vi "fun_Adjust waveform t0.vi"(8 "error in (no error)":errorcluster, 9 "delta Timestamp(ticks)":u64, 10 "waveform (Y)":waveform(dbl)[](array[waveform]), 11 "Handle In":T1 {"Handle" format="0x%08x"; "Conn" format="0x%08x"}) -> (0 "error out":errorcluster, 2 "Adjusted Waveform":waveform(dbl)[](array[waveform]), 3 "Handle Out":T1 {"Handle" format="0x%08x"; "Conn" format="0x%08x"})   [LabVIEW 2016]
uses:
  <instrlib>/Zurich Instruments LabOne/Public/ziTypeHandle.ctl
  <instrlib>/Zurich Instruments LabOne/Public/Utility/ziTicksToS_single.vi
  <instrlib>/Zurich Instruments LabOne/Zurich Instruments LabOne.lvlib
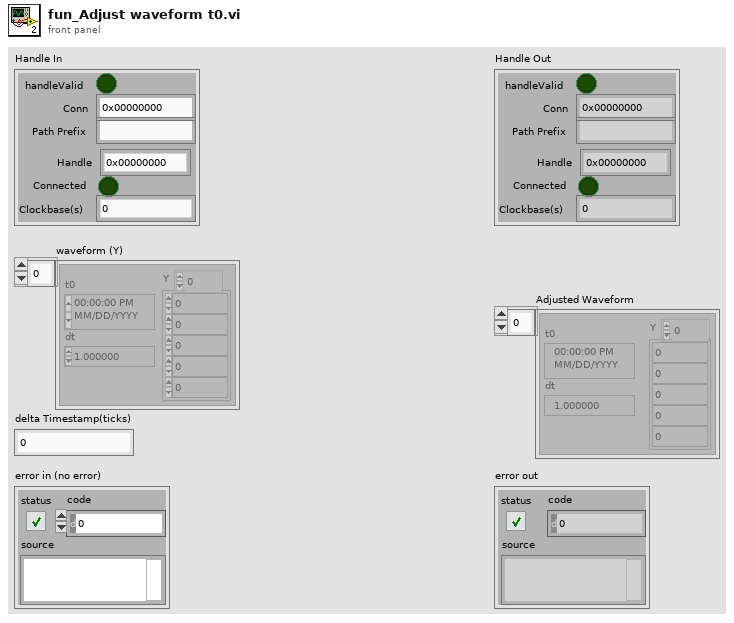
[diagram p1: front panel]
types:
  T1 = typedef "Zurich Instruments LabOne.lvlib/ziTypeHandle.ctl" = cluster{"handleValid":bool, "Conn":u64, "Path Prefix":string, "Handle":u64, "Connected":bool, "Clockbase(s)":dbl}
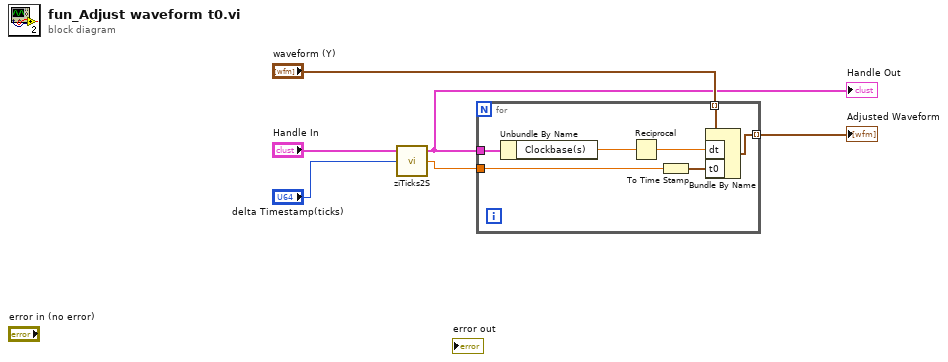
[diagram p0: block diagram]
diagram:
  n1 = call-poly <instrlib>:"ziTicks2S.vi"("Timestamp(ticks)"="delta Timestamp(ticks)", "Handle In"="Handle In") -> ("Timestamp(s)"=w1:dbl, "Handle Out"=w3:T1)  [unwired: 1 in, 1 out]
  "Handle Out" <- w3
  n2 = for {
    tunnel: "waveform (Y)" -> [w13] mode=indexing
    tunnel: [w12] -> w6 mode=indexing
    tunnel: w3 -> [w9]
    tunnel: w1 -> [w7]
    n3 = Unbundle By Name(w9) -> ("Clockbase(s)"=w11:dbl)
    n4 = Reciprocal(x=w11) -> (1/x=w10:dbl)
    n5 = To Time Stamp(1:w7) -> (0:w8:timestamp)
    n6 = Bundle By Name(cluster=w13, "dt"=w10, "t0"=w8) -> (w12:waveform(dbl))
  }
  "Adjusted Waveform" <- w6
